vi "create_command_string.vi"(7 "Kp":dbl, 8 "Error In":errorcluster, 9 "SP":dbl, 10 "Kd":dbl, 11 "Ki":dbl) -> (0 "Error Out":errorcluster, 3 "concatenated string":string)   [LabVIEW 2019]
doc: "Create a command string based on the gains and setpoint input."
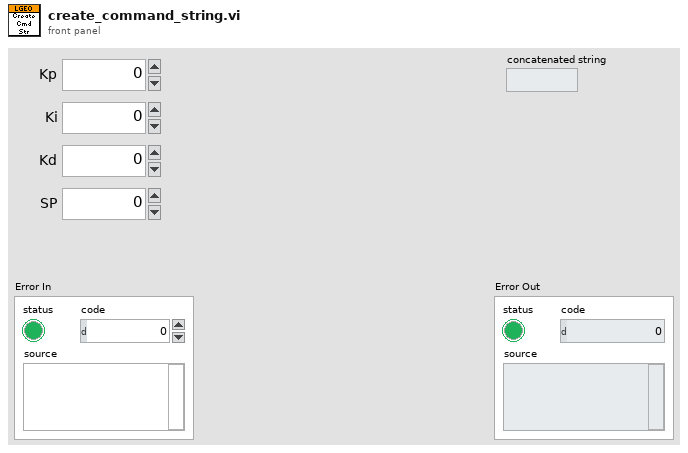
[diagram p1: front panel]
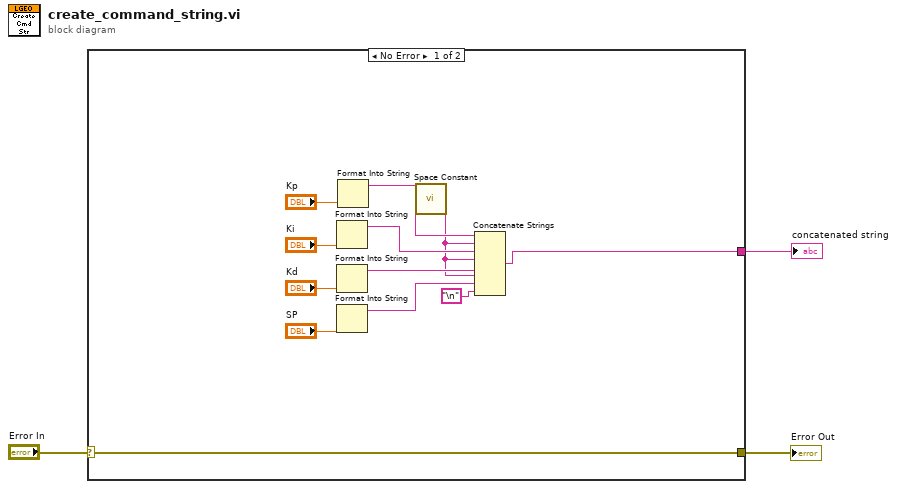
[diagram p0: block diagram]
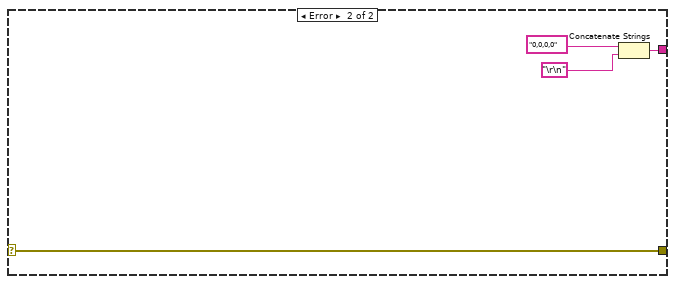
[diagram p2: hidden frame]
diagram:
  n1 = case shown="No Error" "Error In" {
    selector: "Error In" -> [w7 w19]
    tunnel: [w7 w19] -> w2
    tunnel: [w6 w18] -> w1
    frame No Error {
      n2 = Format Into String("Ki") -> (resulting string=w10:string)  [unwired: 3 in, 1 out]
      n3 = Format Into String("Kd") -> (resulting string=w9:string)  [unwired: 3 in, 1 out]
      n4 = Format Into String("SP") -> (resulting string=w8:string)  [unwired: 3 in, 1 out]
      n5 = Format Into String("Kp") -> (resulting string=w14:string)  [unwired: 3 in, 1 out]
      n6 = call <vilib>:"Space Constant.vi"() -> ("String"=w5:string)
      n7 = Concatenate Strings(w14, w5, w10, w5, w9, w5, w8, "\n") -> (w6:string)
    }
    frame Error {
      n8 = Concatenate Strings("0,0,0,0", "\r\n") -> (w18:string)
    }
  }
  "Error Out" <- w2
  "concatenated string" <- w1
